vi "RCV CAN data.vi"() -> ()   [LabVIEW 2020, in "PCANBasic.lvlib"]
uses:
  <userlib>/PCAN Basic/PCANBasic.lvlib
  <userlib>/PCAN Basic/Controls/Channel.ctl
  <userlib>/PCAN Basic/Controls/BaudrateEenum.ctl
  <userlib>/PCAN Basic/Controls/CAN MSG Cluster.ctl
  <userlib>/PCAN Basic/Controls/Timestampbuffer.ctl
  <userlib>/PCAN Basic/Controls/Parameter.ctl
  <vilib>/Platform/TimedLoop/XDataNode/timing_clust.ctl
  <vilib>/Platform/TimedLoop/XDataNode/nitl_modes.ctl
  <vilib>/Platform/TimedLoop/XDataNode/wakeup.ctl
  <userlib>/PCAN Basic/VIs/Get Value/PCAN Get CHANNEL CONDITION.vi
  <vilib>/Platform/TimedLoop/XDataNode/XDataNode.xnode
  <vilib>/Platform/TimedLoop/XDataNode/XDNodeRunTimeDep.lvlib
panel:
  out "CAN Timestamp":T1[](array[typedef])
  out "CAN Data":T2[](array[typedef]) {"ID" format="%.0x"}
  in  "Release all channels first":bool=TRUE
  in  "BTR0BTR1":T3
  in  "Channel":T4=enum."PCAN_USBBUS1"
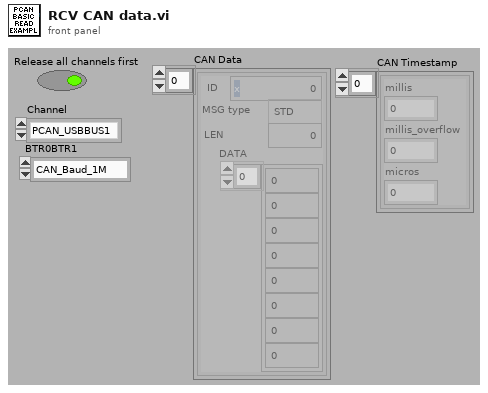
[diagram p1: front panel]
types:
  T1 = typedef "PCANBasic.lvlib/Timestampbuffer.ctl" = cluster{"millis":u32, "millis_overflow":u16, "micros":u16}
  T2 = typedef "PCANBasic.lvlib/CAN MSG Cluster.ctl" = cluster{"ID":u32, "MSG type":enum8{"STD", "RTR", "XTD", "XTD RTR", "STATUS"}, "LEN":i8, "DATA":u8[]}
  T3 = typedef "PCANBasic.lvlib/BaudrateEenum.ctl" = enum16{"CAN_Baud_1M", "CAN_Baud_800K", "CAN_BAUD_500K", "CAN_BAUD_250K", "CAN_BAUD_125K", "CAN_BAUD_100K", "CAN_BAUD_95K", "CAN_BAUD_83K", "CAN_BAUD_50K", "CAN_BAUD_47K", "CAN_BAUD_33K", "CAN_BAUD_20K", "CAN_BAUD_10K", "CAN_BAUD_5K", "User Baudrate"}
  T4 = typedef "PCANBasic.lvlib/Channel.ctl" = enum16{"PCAN_NONEBUS", "not used1", "not used2", "not used3", "not used4", "not used5", "not used6", "not used7", "not used8", "not used9", "not used10", "not used11", "not used12", "not used13", "not used14", "not used15", "not used16", "not used17", "not used18", "not used19", "not used20", "not used21", "not used22", "not used23", "not used24", "not used25", "not used26", "not used27", "not used28", "not used29", "not used30", "not used31", "not used32", "PCAN_ISABUS1", "PCAN_ISABUS2", "PCAN_ISABUS3", "PCAN_ISABUS4", "PCAN_ISABUS5", "PCAN_ISABUS6", "PCAN_ISABUS7", "PCAN_ISABUS8", "not used41", "not used42", "not used43", "not used44", "not used45", "not used46", "not used47", "not used48", "PCAN_DNGBUS1", "not used50", "not used51", "not used52", "not used53", "not used54", "not used55", "not used56", "not used57", "not used58", "not used59", "not used60", "not used61", "not used62", "not used63", "not used64", "PCAN_PCIBUS1", "PCAN_PCIBUS2", "PCAN_PCIBUS3", "PCAN_PCIBUS4", "PCAN_PCIBUS5", "PCAN_PCIBUS6", "PCAN_PCIBUS7", "PCAN_PCIBUS8", "not used73", "not used74", "not used75", "not used76", "not used77", "not used78", "not used79", "not used80", "PCAN_USBBUS1", "PCAN_USBBUS2", "PCAN_USBBUS3", "PCAN_USBBUS4", "PCAN_USBBUS5", "PCAN_USBBUS6", "PCAN_USBBUS7", "PCAN_USBBUS8", "Not used89", "Not used90", "Not used91", "Not used92", "Not used93", "Not used94", "Not used95", "Not used96", "PCAN_PCCBUS1", "PCAN_PCCBUS2"}
  T5 = typedef "PCANBasic.lvlib/Parameter.ctl" = enum16{"Not Available", "PCAN device number", "PCAN 5-volt power", "PCAN receive event", "PCAN message filter", "PCAN API version", "PCAN channel version", "PCAN bus-off auto reset", "PCAN listen-only", "PCAN log location", "PCAN log status", "PCAN log configure", "PCAN log text", "PCAN channel condition", "PCAN hardware name"}
  T6 = typedef "PCANBasic.lvlib/Channel Availability.ctl" = enum16{"PCAN_CHANNEL_UNAVAILABLE", "PCAN_CHANNEL_AVAILABLE ", "PCAN_CHANNEL_OCCUPIED "}
  T7 = typedef "XDNodeRunTimeDep.lvlib/timing_clust.ctl" = cluster{"Expected End [f-1]":u64, "Actual End [f-1]":u64, "Finished Late? [f-1]":bool, "Expected End [i-1]":u64, "Actual End [i-1]":u64, "Finished Late? [i-1]":bool, "Expected Start [i]":u64, "Actual Start [i]":u64, "Expected Start [f]":u64, "Actual Start [f]":u64, "Source Name":string, "Structure Name":string, "Period":i64, "Deadline":i64, "Offset":i64, "Start":i64, "Priority":i32, "Timeout":i32, "Mode":T8, "Wakeup Reason":T9, "Error":errorcluster, "Source Type":string, "Secondary Source Type":string, "Global End Time":u64, "Global Start Time":u64, "Frame Duration":u64, "Iteration Duration":u64, "Assigned CPU":i32, "I/O Scan Engine Mode":u32}
  T8 = typedef "XDNodeRunTimeDep.lvlib/nitl_modes.ctl" = enum32{"No Change", "Process missed periods, maintain original phase", "Discard missed periods, maintain original phase", "Process missed periods, ignore original phase", "Discard missed periods, ignore original phase"}
  T9 = typedef "XDNodeRunTimeDep.lvlib/wakeup.ctl" = enum32{"Normal", "Aborted", "Asynchronous wakeup", "Timing source error", "Timed loop error", "Timeout"}
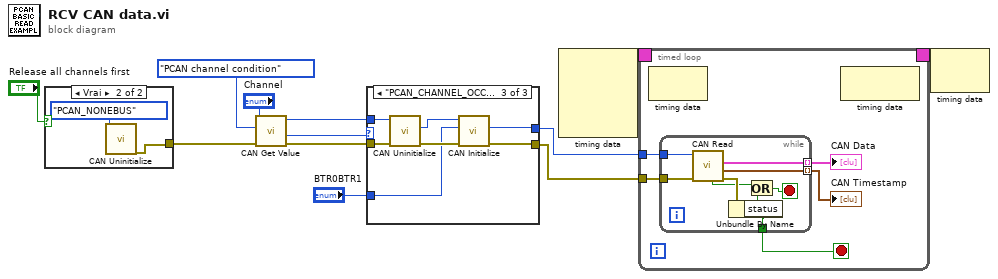
[diagram p0: block diagram]
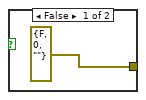
[diagram p2: hidden frame]
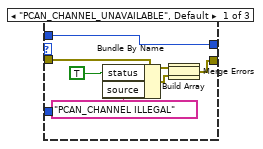
[diagram p3: hidden frame]
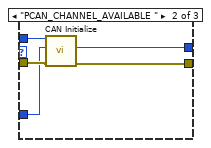
[diagram p4: hidden frame]
diagram:
  n1 = case shown="Vrai" "Release all channels first" {
    tunnel: [errorcluster {"status"=FALSE, "code"=0, "source"=""} ("error out") w15] -> w6
    frame False {
    }
    frame True {
      n2 = call <userlib>:"CAN Uninitialize.vi"("Channel"=Channel."PCAN_NONEBUS") -> ("error out"=w15:errorcluster)  [unwired: 8 in, 2 out]
    }
  }
  n3 = call-poly <userlib>:"CAN Get Value.vi"("error in (no error)"=w6, "Parameter"=Parameter."PCAN channel condition", "Channel"="Channel") -> ("error out"=w9:errorcluster, "Channel condition"=w8:T6, "Channel out"=w10:T4)  [unwired: 6 in]
  n4 = case shown="\"PCAN_CHANNEL_OCCUPIED \"" w8 {
    tunnel: [w21 w27 w29] -> w1
    tunnel: w10 -> [w22 w26 w33]
    tunnel: w9 -> [w20 w25 w34]
    tunnel: "BTR0BTR1" -> [_ w24 w30]
    tunnel: [w22 w23 w28] -> w2
    frame "PCAN_CHANNEL_UNAVAILABLE", Default {
      n5 = Bundle By Name(cluster=w20, "status"=TRUE, "source"="PCAN_CHANNEL ILLEGAL") -> (w17:errorcluster)
      n6 = Build Array(w20, w17) -> (w16:errorcluster[])
      n7 = Merge Errors(w16) -> (w21:errorcluster)
    }
    frame "PCAN_CHANNEL_AVAILABLE " {
      n8 = call <userlib>:"CAN Initialize.vi"("error in (no error)"=w25, "BTR0BTR1"=w24, "Channel"=w26) -> ("error out"=w27:errorcluster, "Channel out"=w23:T4)  [unwired: 6 in, 1 out]
    }
    frame "PCAN_CHANNEL_OCCUPIED " {
      n9 = call <userlib>:"CAN Uninitialize.vi"("error in (no error)"=w34, "Channel"=w33) -> ("error out"=w32:errorcluster, "Channel out"=w31:T4)  [unwired: 7 in, 1 out]
      n10 = call <userlib>:"CAN Initialize.vi"("error in (no error)"=w32, "BTR0BTR1"=w30, "Channel"=w31) -> ("error out"=w29:errorcluster, "Channel out"=w28:T4)  [unwired: 6 in, 1 out]
    }
  }
  n11 = node-c288() -> (w4:T7)  [unwired: 4 in]
  n12 = timed-loop {
    timing: w4 -> [_]
    timing-out: [_] -> w3
    tunnel: w2 -> [w39]
    tunnel: w1 -> [w38]
    stop <- w37 stop-if-true
    n13 = node-c288() -> ()  [unwired: 1 in, 1 out]
    n14 = while {
      tunnel: w39 -> [w47]
      tunnel: w38 -> [w46]
      tunnel: [w43] -> w37
      tunnel: [w42] -> w35 mode=indexing
      tunnel: [w40] -> w36 mode=indexing
      stop <- w44 stop-if-true
      n15 = call <userlib>:"CAN Read.vi"("error in (no error)"=w46, "Channel"=w47) -> ("error out"=w45:errorcluster, "TimestampBuffer out"=w42:T1, "CAN_Message out"=w40:T2, "rcv queue empty"=w41:bool)  [unwired: 5 in, 1 out]
      n16 = Unbundle By Name(w45) -> ("status"=w43:bool)
      n17 = Or(x=w41, y=w43) -> (x .or. y?=w44:bool)
    }
    "CAN Data" <- w36
    "CAN Timestamp" <- w35
    n18 = node-c288() -> ()  [unwired: 1 in, 1 out]
  }
  n19 = node-c288(w3) -> ()  [unwired: 1 out]
